vi "FTW-Endpoint-Listen.vi"(0 "FTW Endpoint":refnum<class "FTW-Endpoint-TCP.lvclass">, 11 "error in":errorcluster) -> (4 "FTW Endpoint out":refnum<class "FTW-Endpoint-TCP.lvclass">, 6 "New Connection":refnum<class "FTW-Endpoint.lvclass">, 15 "error out":errorcluster)   [LabVIEW 2015, in "FTW-Endpoint-TCP.lvclass"]
uses:
  FTW-Endpoint-TCP.lvclass
  Endpoint/FTW-Endpoint.lvclass
  FTW-Endpoint-TCP.lvclass/FTW-Endpoint-TCP.ctl
panel:
  # "Inputs"
  # "Outputs"
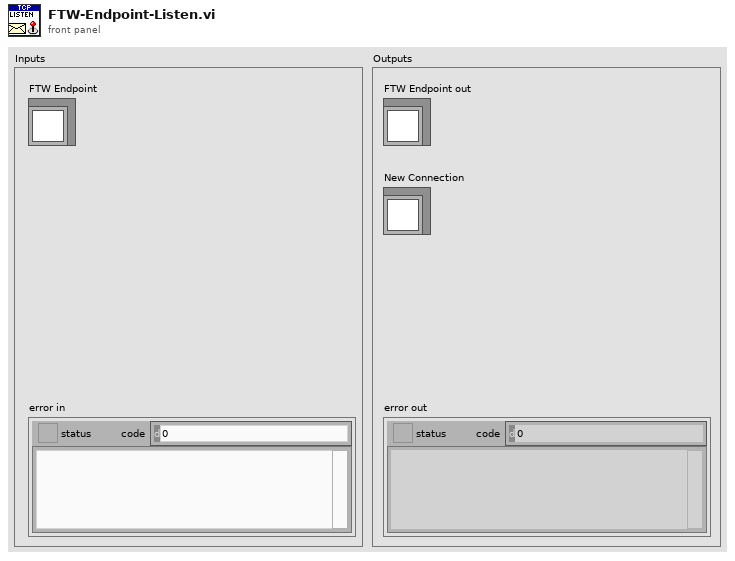
[diagram p1: front panel]
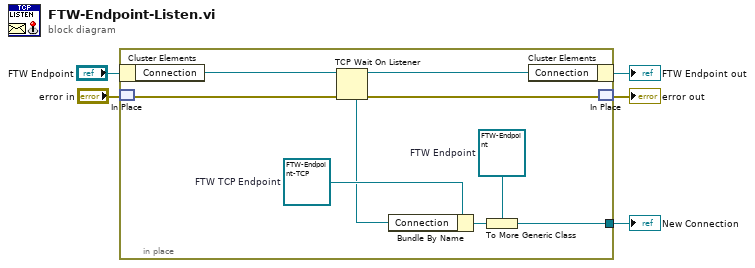
[diagram p0: block diagram]
diagram:
  n1 = in-place {
    in-place-border: [w9] -> w1
    w8 = refnum<class "FTW-Endpoint-TCP.lvclass"> refnum  # FTW TCP Endpoint
    w10 = refnum<class "FTW-Endpoint.lvclass"> refnum  # FTW Endpoint
    n2 = in-place-cluster #1("FTW Endpoint") -> ("Connection"=w12:refnum<k5>)
    n3 = in-place-match #2("error in") -> (w14:errorcluster)
    n4 = TCP Wait On Listener(8:w14, 11:w12) -> (0:w13:errorcluster, 3:w11:refnum<k5>, 4:w6:refnum<k5>)  [unwired: 2 in, 2 out]
    n5 = Bundle By Name(cluster=w8, "Connection"=w6) -> (w7:refnum<class "FTW-Endpoint-TCP.lvclass">)
    n6 = To More Generic Class(target class=w10, reference=w7) -> (generic class reference=w9:refnum<class "FTW-Endpoint.lvclass">)
    n7 = in-place-cluster #1("Connection"=w11) -> (→"FTW Endpoint out":refnum<class "FTW-Endpoint-TCP.lvclass">)
    n8 = in-place-match #2(w13) -> (→"error out":errorcluster)
  }
  "New Connection" <- w1
